vi "5492_SwitchAutoLeft1Cube.vi"(11 "Side":string) -> ()   [LabVIEW 2017]
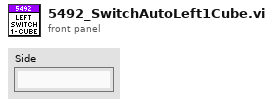
[diagram p1: front panel]
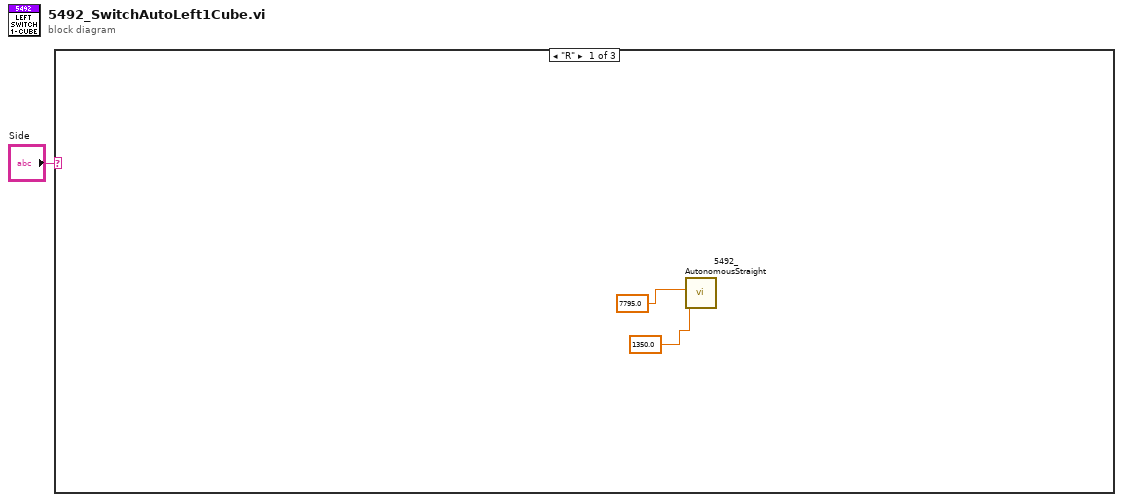
[diagram p0: block diagram]
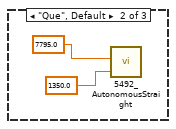
[diagram p2: hidden frame]
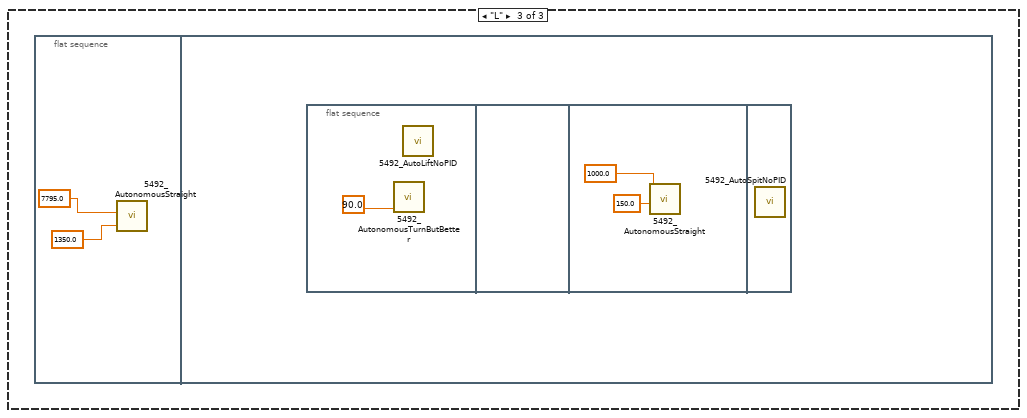
[diagram p3: hidden frame]
diagram:
  n1 = case shown="\"R\"" "Side" {
    frame "R" {
      n2 = call "5492_AutonomousStraight.vi"("Length"=1350.0, "Position Goal"=7795.0) -> ()  [unwired: 9 in, 1 out]
    }
    frame "Que", Default {
      n3 = call "5492_AutonomousStraight.vi"("Length"=1350.0, "Position Goal"=7795.0) -> ()  [unwired: 9 in, 1 out]
    }
    frame "L" {
      n4 = flat-sequence {
        frame #0 {
          n5 = call "5492_AutonomousStraight.vi"("Length"=1350.0, "Position Goal"=7795.0) -> ()  [unwired: 9 in, 1 out]
        }
        frame #1 {
          n6 = flat-sequence {
            frame #0 {
              n7 = call "5492_AutonomousTurnButBetter.vi"("Yaw Goallll"=90.0) -> ()  [unwired: 10 in, 1 out]
              n8 = call "5492_AutoLiftNoPID.vi"() -> ()  [unwired: 12 in]
            }
            frame #1 {
            }
            frame #2 {
              n9 = call "5492_AutonomousStraight.vi"("Length"=150.0, "Position Goal"=1000.0) -> ()  [unwired: 9 in, 1 out]
            }
            frame #3 {
              n10 = call "5492_AutoSpitNoPID.vi"() -> ()  [unwired: 12 in]
            }
          }
        }
      }
    }
  }
